vi "Magnetometer - Heading Case Str_SubVI.vi"(11 "Heading Input (deg)":dbl) -> (3 "Heading Output (Str)":T1)   [LabVIEW 2021]
uses:
  Lab 5/Lab 5 Code/Heading_TDef.ctl
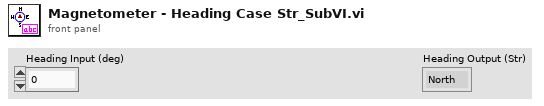
[diagram p1: front panel]
types:
  T1 = typedef "Heading_TDef.ctl" = enum16{"North ", "North East", "East", "Southeast", "South", "Southwest", "West", "Northwest"}
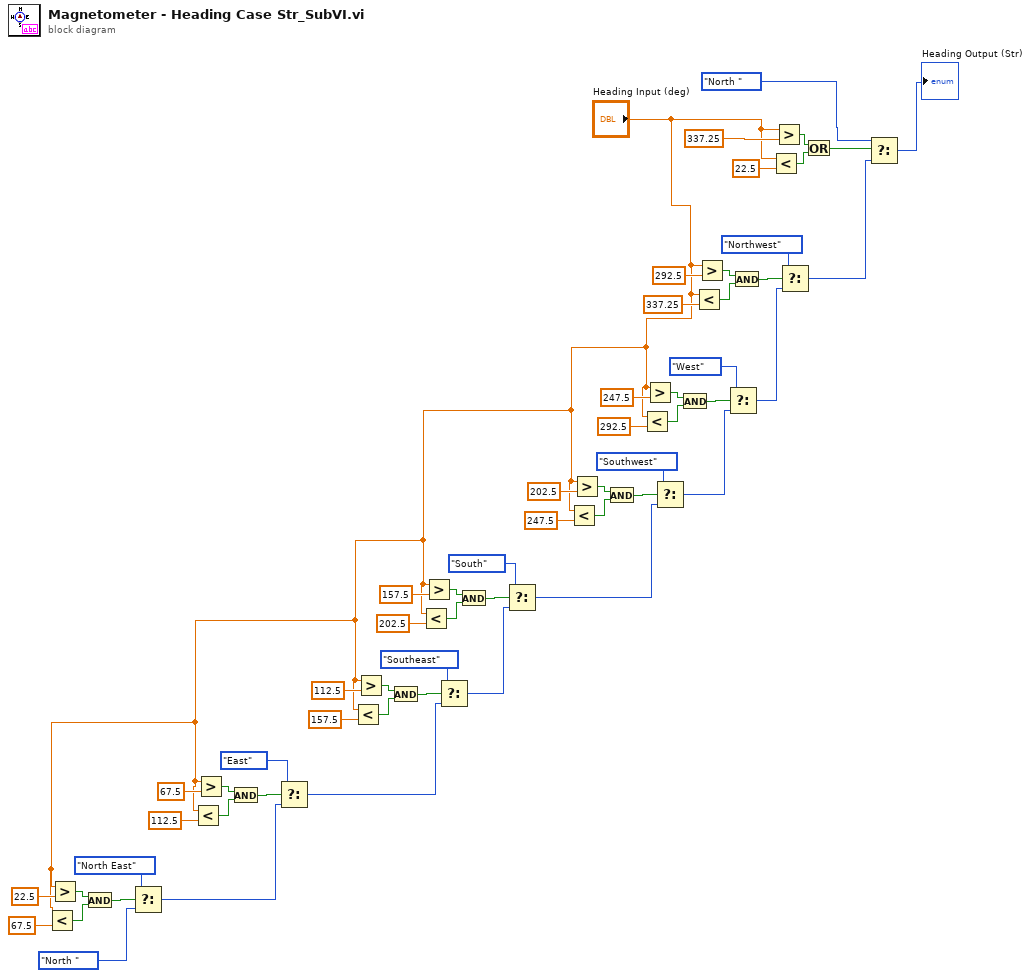
[diagram p0: block diagram]
diagram:
  n1 = Less?(x="Heading Input (deg)", y=67.5) -> (x < y?=w10:bool)
  n2 = Greater?(x="Heading Input (deg)", y=22.5) -> (0:w11:bool)
  n3 = And(x=w11, y=w10) -> (x .and. y?=w9:bool)
  n4 = Select(t=Heading_TDef."North East", s=w9, f=Heading_TDef."North ") -> (s? t:f=w6:T1)
  n5 = Less?(x="Heading Input (deg)", y=112.5) -> (x < y?=w17:bool)
  n6 = Greater?(x="Heading Input (deg)", y=67.5) -> (0:w16:bool)
  n7 = And(x=w16, y=w17) -> (x .and. y?=w18:bool)
  n8 = Select(t=Heading_TDef."East", s=w18, f=w6) -> (s? t:f=w4:T1)
  n9 = Less?(x="Heading Input (deg)", y=157.5) -> (x < y?=w22:bool)
  n10 = Greater?(x="Heading Input (deg)", y=112.5) -> (0:w23:bool)
  n11 = And(x=w23, y=w22) -> (x .and. y?=w21:bool)
  n12 = Less?(x="Heading Input (deg)", y=202.5) -> (x < y?=w29:bool)
  n13 = Greater?(x="Heading Input (deg)", y=157.5) -> (0:w28:bool)
  n14 = Select(t=Heading_TDef."Southeast", s=w21, f=w4) -> (s? t:f=w3:T1)
  n15 = And(x=w28, y=w29) -> (x .and. y?=w30:bool)
  n16 = Select(t=Heading_TDef."South", s=w30, f=w3) -> (s? t:f=w2:T1)
  n17 = Less?(x="Heading Input (deg)", y=247.5) -> (x < y?=w34:bool)
  n18 = Greater?(x="Heading Input (deg)", y=202.5) -> (0:w35:bool)
  n19 = And(x=w35, y=w34) -> (x .and. y?=w33:bool)
  n20 = Less?(x="Heading Input (deg)", y=292.5) -> (x < y?=w43:bool)
  n21 = Greater?(x="Heading Input (deg)", y=247.5) -> (0:w42:bool)
  n22 = Select(t=Heading_TDef."Southwest", s=w33, f=w2) -> (s? t:f=w1:T1)
  n23 = And(x=w42, y=w43) -> (x .and. y?=w44:bool)
  n24 = Less?(x="Heading Input (deg)", y=337.25) -> (x < y?=w48:bool)
  n25 = Greater?(x="Heading Input (deg)", y=292.5) -> (0:w49:bool)
  n26 = Select(t=Heading_TDef."West", s=w44, f=w1) -> (s? t:f=w38:T1)
  n27 = And(x=w49, y=w48) -> (x .and. y?=w47:bool)
  n28 = Less?(x="Heading Input (deg)", y=22.5) -> (x < y?=w54:bool)
  n29 = Greater?(x="Heading Input (deg)", y=337.25) -> (0:w55:bool)
  n30 = Select(t=Heading_TDef."Northwest", s=w47, f=w38) -> (s? t:f=w39:T1)
  n31 = Or(x=w55, y=w54) -> (x .or. y?=w56:bool)
  n32 = Select(t=Heading_TDef."North ", s=w56, f=w39) -> (s? t:f=→"Heading Output (Str)":T1)
